vi "Inverse Error Function_Estimation.vi"(11 "x":dbl) -> (3 "erf^-1(x)":dbl)   [LabVIEW 2017, in "NI_AAL_MathFunc.lvlib"]
uses:
  <vilib>/gmath/NI_AAL_MathFunc.lvlib
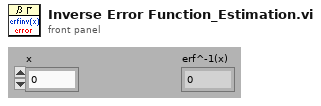
[diagram p1: front panel]
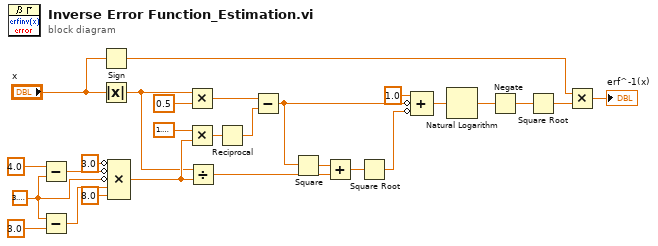
[diagram p0: block diagram]
diagram:
  w24 = 3.141592653589793
  n1 = Subtract(x=4.0 ("y"), y=w24) -> (x-y=w25:dbl)
  n2 = Subtract(x=w24, y=3.0) -> (x-y=w23:dbl)
  n3 = Sign(1:"x") -> (0:w2:dbl)
  n4 = Absolute Value(x="x") -> (abs(x)=w4:dbl)
  n5 = Compound Arithmetic op=MULTIPLY(invert 3.0 ("value"), invert w25, invert w24, w23, 8.0 ("value")) -> (w15:dbl)
  n6 = Multiply(x=w4, y=0.5) -> (x*y=w17:dbl)
  n7 = Multiply(x=1.5707963267948966, y=w15) -> (x*y=w18:dbl)
  n8 = Divide(x=w4, y=w15) -> (x/y=w13:dbl)
  n9 = Reciprocal(x=w18) -> (1/x=w16:dbl)
  n10 = Subtract(x=w17, y=w16) -> (x-y=w10:dbl)
  n11 = Square(x=w10) -> (x^2=w14:dbl)
  n12 = Add(x=w14, y=w13) -> (x+y=w12:dbl)
  n13 = Square Root(x=w12) -> (sqrt(x)=w11:dbl)
  n14 = Compound Arithmetic op=ADD(1.0 ("value"), invert w10, invert w11) -> (w8:dbl)
  n15 = Natural Logarithm(1:w8) -> (0:w7:dbl)
  n16 = Negate(x=w7) -> (-x=w6:dbl)
  n17 = Square Root(x=w6) -> (sqrt(x)=w5:dbl)
  n18 = Multiply(x=w2, y=w5) -> (x*y=→"erf^-1(x)":dbl)
